vi "Get Audio In (SubVI).vi"(8 "error in (no error)":errorcluster, 11 "Refnum in":refnum<k20>) -> (0 "error out":errorcluster, 1 "Right Audio In":i16[](array[numeric]), 2 "Left Audio In":i16[](array[numeric]), 3 "Refnum out":refnum<k20>)   [LabVIEW 2016]
uses:
  <vilib>/Utility/error.llb/Error Cluster From Error Code.vi
  <vilib>/rvi/errors/niLvFpgaAdjustHostInterfaceError.vi
  <vilib>/rvi/interface/nirviMethod/nirviMethod.xnode
  <vilib>/FPGAPlugInAG/Dynamic/niLvFpga_ReadFifo_Dynamic.vi
  <vilib>/rvi/errors/niLvFpgaMergeErrorWithErrorCode.vi
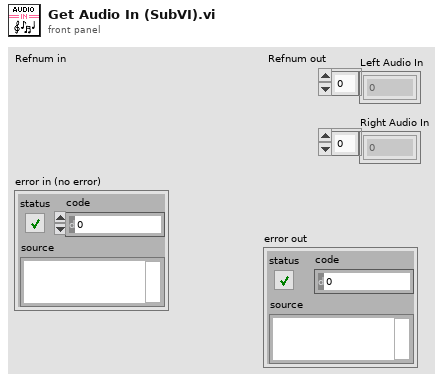
[diagram p1: front panel]
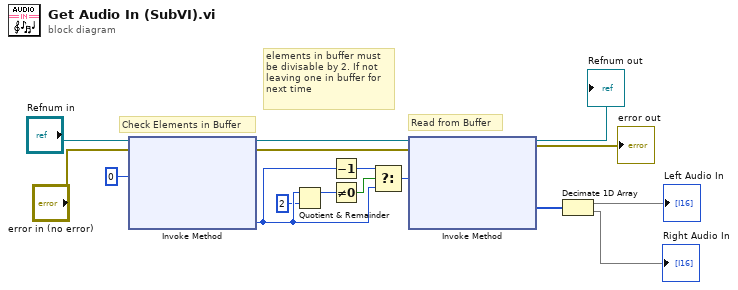
[diagram p0: block diagram]
diagram:
  # "elements in buffer must\nbe divisable by 2. If not\nleaving one in buffer for\nnext time"
  # "Read from Buffer"
  # "Check Elements in Buffer"
  n1 = xnode "Invoke Method"("FPGA VI Reference In"="Refnum in", "error in"="error in (no error)", "Number of Elements"=u32 0) -> ("FPGA VI Reference Out"=w14:refnum<k20>, "error out"=w4:errorcluster, "Elements Remaining"=w9:u32)  [unwired: 1 in, 1 out]
  n2 = Quotient & Remainder(x=w9, y=u32 2) -> (x-y*floor(x/y)=w6:u32)  [unwired: 1 out]
  n3 = Decrement(x=w9) -> (x-1=w8:u32)
  n4 = Not Equal To 0?(x=w6) -> (x != 0?=w7:bool)
  n5 = Select(t=w8, s=w7, f=w9) -> (s? t:f=w10:u32)
  n6 = xnode "Invoke Method"("FPGA VI Reference In"=w14, "error in"=w4, "Number of Elements"=w10) -> ("FPGA VI Reference Out"=→"Refnum out":refnum<k20>, "error out"=→"error out":errorcluster, "Data"=w1:i16[])  [unwired: 1 in, 1 out]
  n7 = Decimate 1D Array(w1) -> (→"Left Audio In":i16[], →"Right Audio In":i16[])
